vi "Get Meta Data.vi"(8 "error in":errorcluster, 11 "UDP in":refnum<class "UDP.lvclass">) -> (0 "error out":errorcluster, 2 "Get Meta Data":T1, 3 "UDP out":refnum<class "UDP.lvclass">)   [LabVIEW 2020, in "Plugin Instrument Driver.lvlib" / "UDP.lvclass"]
doc: "This is a placeholder API to get Meta data details"
uses:
  UDP.lvclass
  builds/Libraries/Shared GUI Library.lvlibp/Shared GUI Library/Device Meta Data Cluster/Get Meta Data.ctl
  Typedefs/Device Details.ctl
  builds/Libraries/Shared GUI Library.lvlibp
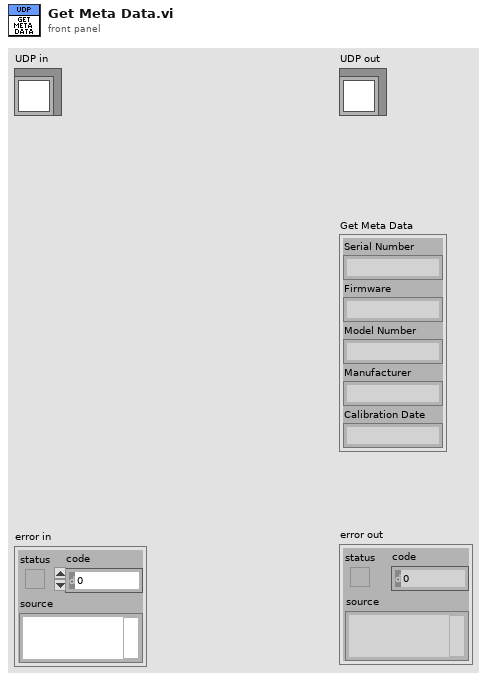
[diagram p1: front panel]
types:
  T1 = typedef "Shared GUI Library.lvlibp/Get Meta Data.ctl" = cluster{"Serial Number":string, "Firmware":string, "Model Number":string, "Manufacturer":string, "Calibration Date":string}
  T2 = typedef "Plugin Instrument Driver.lvlib/UDP.lvclass/Device Details.ctl" = cluster{"Device Port Number":u16, "Device IP":string, "Timeout":i32, "Port Number":u16, "Connection ID":refnum<k16>}
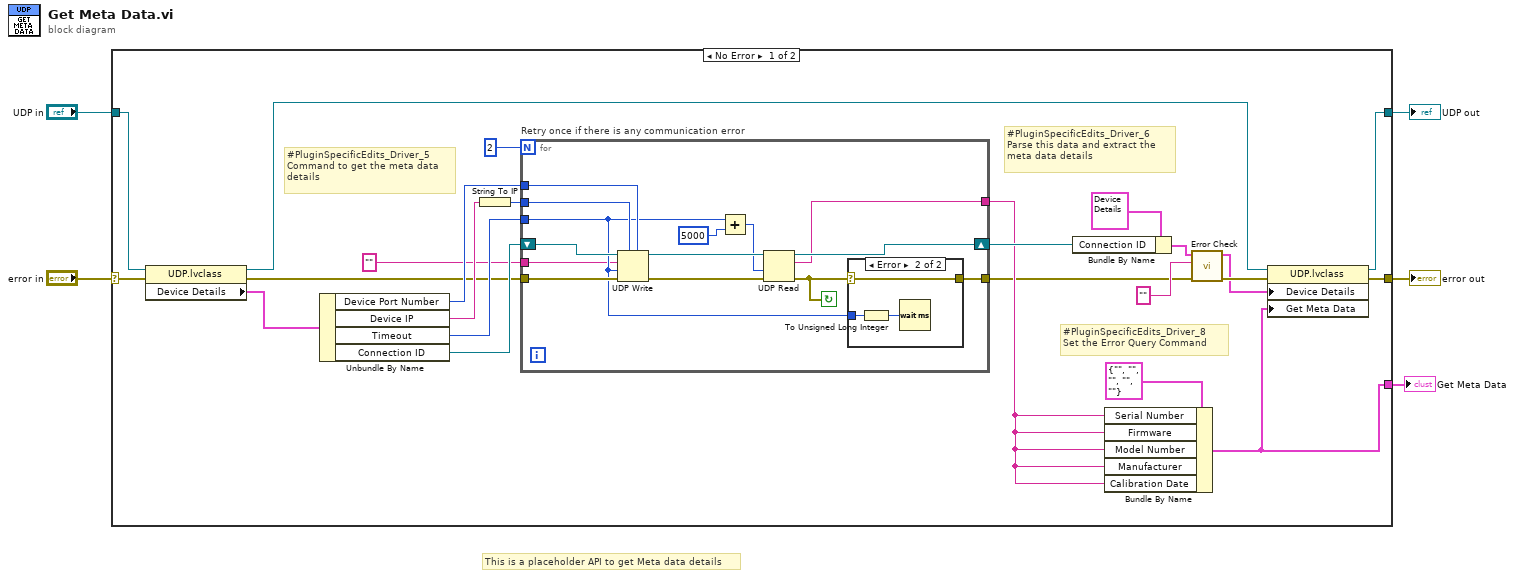
[diagram p0: block diagram]
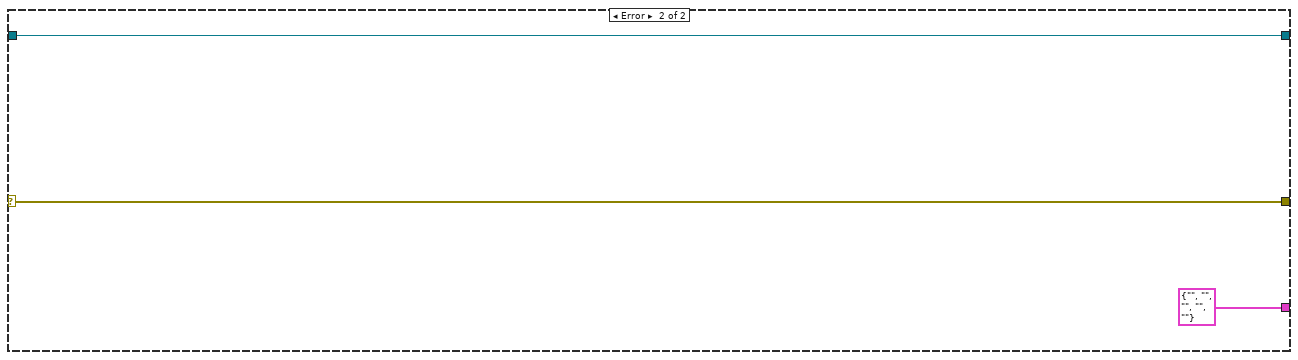
[diagram p3: hidden frame]
diagram:
  # "This is a placeholder API to get Meta data details"
  n1 = case shown="No Error" "error in" {
    selector: "error in" -> [w27 w49]
    tunnel: [w23 w50] -> w3
    tunnel: "UDP in" -> [w24 w50]
    tunnel: [w25 w49] -> w2
    tunnel: [w11 T1 {"Serial Number"="", "Firmware"="", "Model Number"="", "Manufacturer"="", "Calibration Date"=""} ("Get Meta Data")] -> w1
    frame No Error {
      # "#PluginSpecificEdits_Driver_8\nSet the Error Query Command"
      # "#PluginSpecificEdits_Driver_6 \nParse this data and extract the\nmeta data details"
      # "#PluginSpecificEdits_Driver_5 \nCommand to get the meta data\ndetails"
      n2 = property class="UDP.lvclass"(reference=w24, error in=w27) -> (reference out=w26:refnum<class "UDP.lvclass">, error out=w15:errorcluster, "Device Details"=w16:T2)
      n3 = Unbundle By Name(w16) -> ("Device Port Number"=w22:u16, "Device IP"=w21:string, "Timeout"=w20:i32, "Connection ID"=w19:refnum<k16>)
      n4 = String To IP(1:w21) -> (0:w29:u32)
      n5 = for "Retry once if there is any communication error" {
        N: 2 -> [_]
        tunnel: w29 -> [w39]
        tunnel: w22 -> [w38]
        tunnel: [w33] -> w12
        tunnel: w20 -> [w32]
        shift-right: [w41] -> w17
        shift-left: w19 -> [w42]
        tunnel: w15 -> [w43]
        tunnel: [w40] -> w9
        tunnel: "" ("Command") -> [w30]
        stop <- w31 continue-if-true
        n6 = UDP Write(address=w39, port or service name=w38, connection ID=w42, data in=w30, 8:w43, 9:w32) -> (error out=w37:errorcluster, 3:w36:refnum<k16>)
        n7 = Add(x=w32, y=5000) -> (x+y=w35:i32)
        n8 = UDP Read(connection ID=w36, timeout ms (25000)=w35, 8:w37) -> (data out=w33:string, error out=w31:errorcluster, 3:w41:refnum<k16>)  [unwired: 1 in, 2 out]
        n9 = case shown="Error" w31 {
          selector: w31 -> [w44 w47]
          tunnel: [w44 w47] -> w40
          tunnel: w32 -> [_ w46]
          frame No Error {
          }
          frame Error {
            n10 = To Unsigned Long Integer(number=w46) -> (unsigned 32bit integer=w45:u32)
            n11 = Wait (ms)(milliseconds to wait=w45) -> ()  [unwired: 1 out]
          }
        }
      }
      n12 = Bundle By Name(cluster=T2 {"Device Port Number"=2001, "Device IP"="192.168.1.1.100", "Timeout"=5000, "Port Number"=1234, "Connection ID"=refnum} ("Device Details"), "Connection ID"=w17) -> (w6:T2)
      n13 = Bundle By Name(cluster=T1 {"Serial Number"="", "Firmware"="", "Model Number"="", "Manufacturer"="", "Calibration Date"=""} ("Get Meta Data"), "Serial Number"=w12, "Firmware"=w12, "Model Number"=w12, "Manufacturer"=w12, "Calibration Date"=w12) -> (w11:T1)
      n14 = call "Error Check.vi"("error in"=w9, "Error Query Command"="" ("data in"), "Device Details in"=w6) -> ("error out"=w8:errorcluster, "Device Details out"=w7:T2)  [unwired: 7 in]
      n15 = property class="UDP.lvclass"(reference=w26, error in=w8, "Device Details"=w7, "Get Meta Data"=w11) -> (reference out=w23:refnum<class "UDP.lvclass">, error out=w25:errorcluster)
    }
    frame Error {
    }
  }
  "error out" <- w2
  "UDP out" <- w3
  "Get Meta Data" <- w1
